vi "Lab Panel V5.25.vi"() -> ()   [LabVIEW 2017] (continued)
                      frame False {
                        # "update ambient referance temperature"
                        n2219 = case shown="True" w3927 {
                          tunnel: [w3929 100.0] -> w3928
                          frame False {
                            n2220 = local read "TEMP REF cal"() -> (w3929:dbl)
                          }
                          frame True {
                          }
                        }
                        n2221 = disable-structure shown="Disabled" {
                          frame Disabled {
                            n2222 = local read "Temp read loop"() -> ()  [unwired: 1 out]
                          }
                          frame Enabled {
                          }
                        }
                        n2223 = Multiply(x=w3928, y=w3926) -> (x*y=w3925:dbl)
                        n2224 = Subtract(x=w3925, y=272) -> (x-y=w3923:dbl)
                        "Amb Tp" <- w3923
                        n2225 = local write "Ref deg C"(w3923) -> ()
                        "deg C (volts)" <- w3926
                      }
                      frame True {
                      }
                    }
                  }
                }
              }
            }
          }
          frame #13 {
            # "save test data to file"
            n2226 = Get Date/Time In Seconds() -> (seconds since 1Jan1904=w3931:timestamp)
            "File Time Stamp" <- w3931
            n2227 = local read "on loops"() -> (w3950:dbl)
            n2228 = local read "jig cycle"() -> (w3947:dbl)
            n2229 = Format Date/Time String(time format string (%c)="%H:%M%:%S", seconds (now)=w3931) -> (date/time string=w3935:string)  [unwired: 1 in]
            n2230 = Add(x=w3950, y=2) -> (x+y=w3948:dbl)
            n2231 = Build Array(w3935) -> (w3934:string[])
            n2232 = Equal?(x=w3947, y=1) -> (x = y?=w3933:bool)
            n2233 = Equal?(x=w3947, y=w3948) -> (x = y?=w3932:bool)
            n2234 = stacked-sequence {
              tunnel: w3946 -> [w3956 _ _ _ _ _ _ _ _ _]
              tunnel: w3945 -> [_ w4032 _ _ _ _ _ _ _ _]
              tunnel: w3944 -> [_ _ w4112 _ _ _ _ _ _ _]
              tunnel: w3943 -> [_ _ _ w4192 _ _ _ _ _ _]
              tunnel: w3942 -> [_ _ _ _ w4272 _ _ _ _ _]
              tunnel: w3941 -> [_ _ _ _ _ w4352 _ _ _ _]
              tunnel: w3940 -> [_ _ _ _ _ _ w4432 _ _ _]
              tunnel: w3939 -> [_ _ _ _ _ _ _ w4512 _ _]
              tunnel: w3938 -> [_ _ _ _ _ _ _ _ w4592 _]
              tunnel: w3937 -> [_ _ _ _ _ _ _ _ _ w4672]
              tunnel: w3934 -> [w3955 w4036 w4116 w4196 w4276 w4356 w4436 w4516 w4596 w4676]
              tunnel: w3933 -> [w3954 w4035 w4115 w4195 w4275 w4355 w4435 w4515 w4595 w4675]
              tunnel: w3932 -> [w3953 w4034 w4114 w4194 w4274 w4354 w4434 w4514 w4594 w4674]
              tunnel: w3931 -> [w3952 w4033 w4113 w4193 w4273 w4353 w4433 w4513 w4593 w4673]
              frame #0 {
                n2235 = case shown="True" w3956 {
                  tunnel: w3955 -> [_ w3961]
                  tunnel: w3954 -> [_ w3960]
                  tunnel: w3953 -> [_ w3958]
                  tunnel: w3952 -> [_ w3957]
                  frame False {
                  }
                  frame True {
                    n2236 = local read "DISP LAB01-1"() -> (w3962:T4)
                    n2237 = local read "SIG LAB01-1"() -> (w3963:T2)
                    n2238 = local read "ON L01-1"() -> (w3959:cluster{"amps":dbl, "volts":dbl, "pf":dbl})
                    n2239 = Unbundle(w3963) -> ("AMPS"=w3969:dbl, "VOLTS"=w3967:dbl, "PF"=w3966:dbl, "Tmp Live"=w3965:dbl, "Tmp Neut"=w3968:dbl)
                    n2240 = Unbundle(w3962) -> ("CYCLE"=w3964:dbl)  [unwired: 2 out]
                    n2241 = stacked-sequence {
                      tunnel: w3969 -> [w3973 w3992]
                      tunnel: w3968 -> [_ w3991]
                      tunnel: w3967 -> [w3972 w3990]
                      tunnel: w3966 -> [w3971 w3989]
                      tunnel: w3965 -> [_ w3988]
                      tunnel: w3964 -> [_ w3987]
                      tunnel: w3961 -> [_ w3986]
                      tunnel: w3960 -> [w3974 _]
                      tunnel: w3959 -> [w3970 w3984]
                      tunnel: w3958 -> [_ w3985]
                      tunnel: w3957 -> [_ w3980]
                      frame #0 {
                        n2242 = case shown="True" w3974 {
                          tunnel: w3973 -> [_ w3979]
                          tunnel: w3972 -> [_ w3978]
                          tunnel: w3971 -> [_ w3977]
                          tunnel: w3970 -> [_ w3975]
                          frame False {
                          }
                          frame True {
                            n2243 = Bundle(cluster=w3975, "amps"=w3979, "volts"=w3978, "pf"=w3977) -> (w3976:cluster{"amps":dbl, "volts":dbl, "pf":dbl})
                            n2244 = local write "ON L01-1"(w3976) -> ()
                          }
                        }
                      }
                      frame #1 {
                        n2245 = Unbundle(w3984) -> ("amps"=w3983:dbl, "volts"=w3982:dbl, "pf"=w3981:dbl)
                        n2246 = case shown="True" w3985 {
                          tunnel: w3992 -> [_ w3993]
                          tunnel: w3991 -> [_ w4031]
                          tunnel: w3990 -> [_ _]
                          tunnel: w3989 -> [_ _]
                          tunnel: w3988 -> [_ w4030]
                          tunnel: w3987 -> [_ w4029]
                          tunnel: w3986 -> [_ w3997]
                          tunnel: w3983 -> [_ w3994]
                          tunnel: w3982 -> [_ w4026]
                          tunnel: w3981 -> [_ w4025]
                          tunnel: w3980 -> [_ w3995]
                          frame False {
                          }
                          frame True {
                            n2247 = local read "TDMS LAB01-1"() -> (w4028:refnum<k34>)
                            n2248 = Build Array(w4026) -> (w4022:dbl[])
                            n2249 = Build Array(w4025) -> (w4021:dbl[])
                            n2250 = Build Array(w4030) -> (w4020:dbl[])
                            n2251 = Build Array(w4031) -> (w4019:dbl[])
                            n2252 = Build Array(w3994) -> (w4024:dbl[])
                            n2253 = Build Array(w3993) -> (w4023:dbl[])
                            n2254 = Build Array(w4029) -> (w4018:dbl[])
                            n2255 = Build Array("AMPS ON", "AMPS OFF", "VOLTS", "PF", "TEMP Live", "TEMP Neut", "CYCLE") -> (w4002:string[])
                            n2256 = Bundle By Name("Y"=w4024, "t0"=w3995) -> (w4017:waveform(dbl))  [unwired: 1 in]
                            n2257 = Bundle By Name("Y"=w4023, "t0"=w3995) -> (w4016:waveform(dbl))  [unwired: 1 in]
                            n2258 = Bundle By Name("Y"=w4022, "t0"=w3995) -> (w4015:waveform(dbl))  [unwired: 1 in]
                            n2259 = Bundle By Name("Y"=w4021, "t0"=w3995) -> (w4014:waveform(dbl))  [unwired: 1 in]
                            n2260 = Bundle By Name("Y"=w4020, "t0"=w3995) -> (w4013:waveform(dbl))  [unwired: 1 in]
                            n2261 = Bundle By Name("Y"=w4019, "t0"=w3995) -> (w4012:waveform(dbl))  [unwired: 1 in]
                            n2262 = Bundle By Name("Y"=w4018, "t0"=w3995) -> (w4011:waveform(dbl))  [unwired: 1 in]
                            n2263 = Build Array(w4017, w4016, w4015, w4014, w4013, w4012, w4011) -> (w4010:waveform(dbl)[])
                            n2264 = TDMS Write(0:w4028, 5:"TEST VALUES", 7:w4002, 9:w4010) -> (4:w4001:refnum<k34>, 6:w4000:string, 15:w3999:errorcluster)  [unwired: 2 in, 1 out]
                            n2265 = TDMS Write(0:w4001, 5:w4000, 7:"TIME", 9:w3997, 11:w3999) -> (15:w3996:errorcluster)  [unwired: 1 in, 3 out]
                            n2266 = local write "data file error"(w3996) -> ()
                          }
                        }
                      }
                    }
                  }
                }
              }
              frame #1 {
                n2267 = case shown="True" w4032 {
                  tunnel: w4036 -> [_ w4041]
                  tunnel: w4035 -> [_ w4040]
                  tunnel: w4034 -> [_ w4038]
                  tunnel: w4033 -> [_ w4037]
                  frame False {
                  }
                  frame True {
                    n2268 = local read "DISP LAB01-2"() -> (w4042:T4)
                    n2269 = local read "SIG LAB01-2"() -> (w4043:T2)
                    n2270 = local read "ON L01-2"() -> (w4039:cluster{"amps":dbl, "volts":dbl, "pf":dbl})
                    n2271 = Unbundle(w4043) -> ("AMPS"=w4049:dbl, "VOLTS"=w4047:dbl, "PF"=w4046:dbl, "Tmp Live"=w4045:dbl, "Tmp Neut"=w4048:dbl)
                    n2272 = Unbundle(w4042) -> ("CYCLE"=w4044:dbl)  [unwired: 2 out]
                    n2273 = stacked-sequence {
                      tunnel: w4049 -> [w4053 w4072]
                      tunnel: w4048 -> [_ w4071]
                      tunnel: w4047 -> [w4052 w4070]
                      tunnel: w4046 -> [w4051 w4069]
                      tunnel: w4045 -> [_ w4068]
                      tunnel: w4044 -> [_ w4067]
                      tunnel: w4041 -> [_ w4066]
                      tunnel: w4040 -> [w4054 _]
                      tunnel: w4039 -> [w4050 w4064]
                      tunnel: w4038 -> [_ w4065]
                      tunnel: w4037 -> [_ w4060]
                      frame #0 {
                        n2274 = case shown="True" w4054 {
                          tunnel: w4053 -> [_ w4059]
                          tunnel: w4052 -> [_ w4058]
                          tunnel: w4051 -> [_ w4057]
                          tunnel: w4050 -> [_ w4055]
                          frame False {
                          }
                          frame True {
                            n2275 = Bundle(cluster=w4055, "amps"=w4059, "volts"=w4058, "pf"=w4057) -> (w4056:cluster{"amps":dbl, "volts":dbl, "pf":dbl})
                            n2276 = local write "ON L01-2"(w4056) -> ()
                          }
                        }
                      }
                      frame #1 {
                        n2277 = Unbundle(w4064) -> ("amps"=w4063:dbl, "volts"=w4062:dbl, "pf"=w4061:dbl)
                        n2278 = case shown="True" w4065 {
                          tunnel: w4072 -> [_ w4104]
                          tunnel: w4071 -> [_ w4111]
                          tunnel: w4070 -> [_ _]
                          tunnel: w4069 -> [_ _]
                          tunnel: w4068 -> [_ w4110]
                          tunnel: w4067 -> [_ w4109]
                          tunnel: w4066 -> [_ w4074]
                          tunnel: w4063 -> [_ w4106]
                          tunnel: w4062 -> [_ w4105]
                          tunnel: w4061 -> [_ w4103]
                          tunnel: w4060 -> [_ w4095]
                          frame False {
                          }
                          frame True {
                            n2279 = local read "TDMS LAB01-2"() -> (w4108:refnum<k34>)
                            n2280 = Build Array(w4105) -> (w4100:dbl[])
                            n2281 = Build Array(w4103) -> (w4099:dbl[])
                            n2282 = Build Array(w4110) -> (w4098:dbl[])
                            n2283 = Build Array(w4111) -> (w4097:dbl[])
                            n2284 = Build Array(w4106) -> (w4102:dbl[])
                            n2285 = Build Array(w4104) -> (w4101:dbl[])
                            n2286 = Build Array(w4109) -> (w4096:dbl[])
                            n2287 = Build Array("AMPS ON", "AMPS OFF", "VOLTS", "PF", "TEMP Live", "TEMP Neut", "CYCLE") -> (w4079:string[])
                            n2288 = Bundle By Name("Y"=w4102, "t0"=w4095) -> (w4094:waveform(dbl))  [unwired: 1 in]
                            n2289 = Bundle By Name("Y"=w4101, "t0"=w4095) -> (w4093:waveform(dbl))  [unwired: 1 in]
                            n2290 = Bundle By Name("Y"=w4100, "t0"=w4095) -> (w4092:waveform(dbl))  [unwired: 1 in]
                            n2291 = Bundle By Name("Y"=w4099, "t0"=w4095) -> (w4091:waveform(dbl))  [unwired: 1 in]
                            n2292 = Bundle By Name("Y"=w4098, "t0"=w4095) -> (w4090:waveform(dbl))  [unwired: 1 in]
                            n2293 = Bundle By Name("Y"=w4097, "t0"=w4095) -> (w4089:waveform(dbl))  [unwired: 1 in]
                            n2294 = Bundle By Name("Y"=w4096, "t0"=w4095) -> (w4088:waveform(dbl))  [unwired: 1 in]
                            n2295 = Build Array(w4094, w4093, w4092, w4091, w4090, w4089, w4088) -> (w4087:waveform(dbl)[])
                            n2296 = TDMS Write(0:w4108, 5:"TEST VALUES", 7:w4079, 9:w4087) -> (4:w4078:refnum<k34>, 6:w4077:string, 15:w4076:errorcluster)  [unwired: 2 in, 1 out]
                            n2297 = TDMS Write(0:w4078, 5:w4077, 7:"TIME", 9:w4074, 11:w4076) -> (15:w4073:errorcluster)  [unwired: 1 in, 3 out]
                            n2298 = local write "data file error"(w4073) -> ()
                          }
                        }
                      }
                    }
                  }
                }
              }
              frame #2 {
                n2299 = case shown="True" w4112 {
                  tunnel: w4116 -> [_ w4121]
                  tunnel: w4115 -> [_ w4120]
                  tunnel: w4114 -> [_ w4118]
                  tunnel: w4113 -> [_ w4117]
                  frame False {
                  }
                  frame True {
                    n2300 = local read "DISP LAB02-1"() -> (w4122:T4)
                    n2301 = local read "SIG LAB02-1"() -> (w4123:T2)
                    n2302 = local read "ON L02-1"() -> (w4119:cluster{"amps":dbl, "volts":dbl, "pf":dbl})
                    n2303 = Unbundle(w4123) -> ("AMPS"=w4129:dbl, "VOLTS"=w4127:dbl, "PF"=w4126:dbl, "Tmp Live"=w4125:dbl, "Tmp Neut"=w4128:dbl)
                    n2304 = Unbundle(w4122) -> ("CYCLE"=w4124:dbl)  [unwired: 2 out]
                    n2305 = stacked-sequence {
                      tunnel: w4129 -> [w4133 w4152]
                      tunnel: w4128 -> [_ w4151]
                      tunnel: w4127 -> [w4132 w4150]
                      tunnel: w4126 -> [w4131 w4149]
                      tunnel: w4125 -> [_ w4148]
                      tunnel: w4124 -> [_ w4147]
                      tunnel: w4121 -> [_ w4146]
                      tunnel: w4120 -> [w4134 _]
                      tunnel: w4119 -> [w4130 w4144]
                      tunnel: w4118 -> [_ w4145]
                      tunnel: w4117 -> [_ w4140]
                      frame #0 {
                        n2306 = case shown="True" w4134 {
                          tunnel: w4133 -> [_ w4139]
                          tunnel: w4132 -> [_ w4138]
                          tunnel: w4131 -> [_ w4137]
                          tunnel: w4130 -> [_ w4135]
                          frame False {
                          }
                          frame True {
                            n2307 = Bundle(cluster=w4135, "amps"=w4139, "volts"=w4138, "pf"=w4137) -> (w4136:cluster{"amps":dbl, "volts":dbl, "pf":dbl})
                            n2308 = local write "ON L02-1"(w4136) -> ()
                          }
                        }
                      }
                      frame #1 {
                        n2309 = Unbundle(w4144) -> ("amps"=w4143:dbl, "volts"=w4142:dbl, "pf"=w4141:dbl)
                        n2310 = case shown="True" w4145 {
                          tunnel: w4152 -> [_ w4184]
                          tunnel: w4151 -> [_ w4191]
                          tunnel: w4150 -> [_ _]
                          tunnel: w4149 -> [_ _]
                          tunnel: w4148 -> [_ w4190]
                          tunnel: w4147 -> [_ w4189]
                          tunnel: w4146 -> [_ w4154]
                          tunnel: w4143 -> [_ w4186]
                          tunnel: w4142 -> [_ w4185]
                          tunnel: w4141 -> [_ w4183]
                          tunnel: w4140 -> [_ w4175]
                          frame False {
                          }
                          frame True {
                            n2311 = local read "TDMS LAB02-1"() -> (w4188:refnum<k34>)
                            n2312 = Build Array(w4185) -> (w4180:dbl[])
                            n2313 = Build Array(w4183) -> (w4179:dbl[])
                            n2314 = Build Array(w4190) -> (w4178:dbl[])
                            n2315 = Build Array(w4191) -> (w4177:dbl[])
                            n2316 = Build Array(w4186) -> (w4182:dbl[])
                            n2317 = Build Array(w4184) -> (w4181:dbl[])
                            n2318 = Build Array(w4189) -> (w4176:dbl[])
                            n2319 = Build Array("AMPS ON", "AMPS OFF", "VOLTS", "PF", "TEMP Live", "TEMP Neut", "CYCLE") -> (w4159:string[])
                            n2320 = Bundle By Name("Y"=w4182, "t0"=w4175) -> (w4174:waveform(dbl))  [unwired: 1 in]
                            n2321 = Bundle By Name("Y"=w4181, "t0"=w4175) -> (w4173:waveform(dbl))  [unwired: 1 in]
                            n2322 = Bundle By Name("Y"=w4180, "t0"=w4175) -> (w4172:waveform(dbl))  [unwired: 1 in]
                            n2323 = Bundle By Name("Y"=w4179, "t0"=w4175) -> (w4171:waveform(dbl))  [unwired: 1 in]
                            n2324 = Bundle By Name("Y"=w4178, "t0"=w4175) -> (w4170:waveform(dbl))  [unwired: 1 in]
                            n2325 = Bundle By Name("Y"=w4177, "t0"=w4175) -> (w4169:waveform(dbl))  [unwired: 1 in]
                            n2326 = Bundle By Name("Y"=w4176, "t0"=w4175) -> (w4168:waveform(dbl))  [unwired: 1 in]
                            n2327 = Build Array(w4174, w4173, w4172, w4171, w4170, w4169, w4168) -> (w4167:waveform(dbl)[])
                            n2328 = TDMS Write(0:w4188, 5:"TEST VALUES", 7:w4159, 9:w4167) -> (4:w4158:refnum<k34>, 6:w4157:string, 15:w4156:errorcluster)  [unwired: 2 in, 1 out]
                            n2329 = TDMS Write(0:w4158, 5:w4157, 7:"TIME", 9:w4154, 11:w4156) -> (15:w4153:errorcluster)  [unwired: 1 in, 3 out]
                            n2330 = local write "data file error"(w4153) -> ()
                          }
                        }
                      }
                    }
                  }
                }
              }
              frame #3 {
                n2331 = case shown="True" w4192 {
                  tunnel: w4196 -> [_ w4201]
                  tunnel: w4195 -> [_ w4200]
                  tunnel: w4194 -> [_ w4198]
                  tunnel: w4193 -> [_ w4197]
                  frame False {
                  }
                  frame True {
                    n2332 = local read "DISP LAB02-2"() -> (w4202:T4)
                    n2333 = local read "SIG LAB02-2"() -> (w4203:T2)
                    n2334 = local read "ON L02-2"() -> (w4199:cluster{"amps":dbl, "volts":dbl, "pf":dbl})
                    n2335 = Unbundle(w4203) -> ("AMPS"=w4209:dbl, "VOLTS"=w4207:dbl, "PF"=w4206:dbl, "Tmp Live"=w4205:dbl, "Tmp Neut"=w4208:dbl)
                    n2336 = Unbundle(w4202) -> ("CYCLE"=w4204:dbl)  [unwired: 2 out]
                    n2337 = stacked-sequence {
                      tunnel: w4209 -> [w4213 w4232]
                      tunnel: w4208 -> [_ w4231]
                      tunnel: w4207 -> [w4212 w4230]
                      tunnel: w4206 -> [w4211 w4229]
                      tunnel: w4205 -> [_ w4228]
                      tunnel: w4204 -> [_ w4227]
                      tunnel: w4201 -> [_ w4226]
                      tunnel: w4200 -> [w4214 _]
                      tunnel: w4199 -> [w4210 w4224]
                      tunnel: w4198 -> [_ w4225]
                      tunnel: w4197 -> [_ w4220]
                      frame #0 {
                        n2338 = case shown="True" w4214 {
                          tunnel: w4213 -> [_ w4219]
                          tunnel: w4212 -> [_ w4218]
                          tunnel: w4211 -> [_ w4217]
                          tunnel: w4210 -> [_ w4215]
                          frame False {
                          }
                          frame True {
                            n2339 = Bundle(cluster=w4215, "amps"=w4219, "volts"=w4218, "pf"=w4217) -> (w4216:cluster{"amps":dbl, "volts":dbl, "pf":dbl})
                            n2340 = local write "ON L02-2"(w4216) -> ()
                          }
                        }
                      }
                      frame #1 {
                        n2341 = Unbundle(w4224) -> ("amps"=w4223:dbl, "volts"=w4222:dbl, "pf"=w4221:dbl)
                        n2342 = case shown="True" w4225 {
                          tunnel: w4232 -> [_ w4264]
                          tunnel: w4231 -> [_ w4271]
                          tunnel: w4230 -> [_ _]
                          tunnel: w4229 -> [_ _]
                          tunnel: w4228 -> [_ w4270]
                          tunnel: w4227 -> [_ w4269]
                          tunnel: w4226 -> [_ w4234]
                          tunnel: w4223 -> [_ w4266]
                          tunnel: w4222 -> [_ w4265]
                          tunnel: w4221 -> [_ w4263]
                          tunnel: w4220 -> [_ w4255]
                          frame False {
                          }
                          frame True {
                            n2343 = local read "TDMS LAB02-2"() -> (w4268:refnum<k34>)
                            n2344 = Build Array(w4265) -> (w4260:dbl[])
                            n2345 = Build Array(w4263) -> (w4259:dbl[])
                            n2346 = Build Array(w4270) -> (w4258:dbl[])
                            n2347 = Build Array(w4271) -> (w4257:dbl[])
                            n2348 = Build Array(w4266) -> (w4262:dbl[])
                            n2349 = Build Array(w4264) -> (w4261:dbl[])
                            n2350 = Build Array(w4269) -> (w4256:dbl[])
                            n2351 = Build Array("AMPS ON", "AMPS OFF", "VOLTS", "PF", "TEMP Live", "TEMP Neut", "CYCLE") -> (w4239:string[])
                            n2352 = Bundle By Name("Y"=w4262, "t0"=w4255) -> (w4254:waveform(dbl))  [unwired: 1 in]
                            n2353 = Bundle By Name("Y"=w4261, "t0"=w4255) -> (w4253:waveform(dbl))  [unwired: 1 in]
                            n2354 = Bundle By Name("Y"=w4260, "t0"=w4255) -> (w4252:waveform(dbl))  [unwired: 1 in]
                            n2355 = Bundle By Name("Y"=w4259, "t0"=w4255) -> (w4251:waveform(dbl))  [unwired: 1 in]
                            n2356 = Bundle By Name("Y"=w4258, "t0"=w4255) -> (w4250:waveform(dbl))  [unwired: 1 in]
                            n2357 = Bundle By Name("Y"=w4257, "t0"=w4255) -> (w4249:waveform(dbl))  [unwired: 1 in]
                            n2358 = Bundle By Name("Y"=w4256, "t0"=w4255) -> (w4248:waveform(dbl))  [unwired: 1 in]
                            n2359 = Build Array(w4254, w4253, w4252, w4251, w4250, w4249, w4248) -> (w4247:waveform(dbl)[])
                            n2360 = TDMS Write(0:w4268, 5:"TEST VALUES", 7:w4239, 9:w4247) -> (4:w4238:refnum<k34>, 6:w4237:string, 15:w4236:errorcluster)  [unwired: 2 in, 1 out]
                            n2361 = TDMS Write(0:w4238, 5:w4237, 7:"TIME", 9:w4234, 11:w4236) -> (15:w4233:errorcluster)  [unwired: 1 in, 3 out]
                            n2362 = local write "data file error"(w4233) -> ()
                          }
                        }
                      }
                    }
                  }
                }
              }
              frame #4 {
                n2363 = case shown="True" w4272 {
                  tunnel: w4276 -> [_ w4281]
                  tunnel: w4275 -> [_ w4280]
                  tunnel: w4274 -> [_ w4278]
                  tunnel: w4273 -> [_ w4277]
                  frame False {
                  }
                  frame True {
                    n2364 = local read "DISP LAB03-1"() -> (w4282:T4)
                    n2365 = local read "SIG LAB03-1"() -> (w4283:T2)
                    n2366 = local read "ON L03-1"() -> (w4279:cluster{"amps":dbl, "volts":dbl, "pf":dbl})
                    n2367 = Unbundle(w4283) -> ("AMPS"=w4289:dbl, "VOLTS"=w4287:dbl, "PF"=w4286:dbl, "Tmp Live"=w4285:dbl, "Tmp Neut"=w4288:dbl)
                    n2368 = Unbundle(w4282) -> ("CYCLE"=w4284:dbl)  [unwired: 2 out]
                    n2369 = stacked-sequence {
                      tunnel: w4289 -> [w4293 w4312]
                      tunnel: w4288 -> [_ w4311]
                      tunnel: w4287 -> [w4292 w4310]
                      tunnel: w4286 -> [w4291 w4309]
                      tunnel: w4285 -> [_ w4308]
                      tunnel: w4284 -> [_ w4307]
                      tunnel: w4281 -> [_ w4306]
                      tunnel: w4280 -> [w4294 _]
                      tunnel: w4279 -> [w4290 w4304]
                      tunnel: w4278 -> [_ w4305]
                      tunnel: w4277 -> [_ w4300]
                      frame #0 {
                        n2370 = case shown="True" w4294 {
                          tunnel: w4293 -> [_ w4299]
                          tunnel: w4292 -> [_ w4298]
                          tunnel: w4291 -> [_ w4297]
                          tunnel: w4290 -> [_ w4295]
                          frame False {
                          }
                          frame True {
                            n2371 = Bundle(cluster=w4295, "amps"=w4299, "volts"=w4298, "pf"=w4297) -> (w4296:cluster{"amps":dbl, "volts":dbl, "pf":dbl})
                            n2372 = local write "ON L03-1"(w4296) -> ()
                          }
                        }
                      }
                      frame #1 {
                        n2373 = Unbundle(w4304) -> ("amps"=w4303:dbl, "volts"=w4302:dbl, "pf"=w4301:dbl)
                        n2374 = case shown="True" w4305 {
                          tunnel: w4312 -> [_ w4344]
                          tunnel: w4311 -> [_ w4351]
                          tunnel: w4310 -> [_ _]
                          tunnel: w4309 -> [_ _]
                          tunnel: w4308 -> [_ w4350]
                          tunnel: w4307 -> [_ w4349]
                          tunnel: w4306 -> [_ w4314]
                          tunnel: w4303 -> [_ w4346]
                          tunnel: w4302 -> [_ w4345]
                          tunnel: w4301 -> [_ w4343]
                          tunnel: w4300 -> [_ w4335]
                          frame False {
                          }
                          frame True {
                            n2375 = local read "TDMS LAB03-1"() -> (w4348:refnum<k34>)
                            n2376 = Build Array(w4345) -> (w4340:dbl[])
                            n2377 = Build Array(w4343) -> (w4339:dbl[])
                            n2378 = Build Array(w4350) -> (w4338:dbl[])
                            n2379 = Build Array(w4351) -> (w4337:dbl[])
                            n2380 = Build Array(w4346) -> (w4342:dbl[])
                            n2381 = Build Array(w4344) -> (w4341:dbl[])
                            n2382 = Build Array(w4349) -> (w4336:dbl[])
                            n2383 = Build Array("AMPS ON", "AMPS OFF", "VOLTS", "PF", "TEMP Live", "TEMP Neut", "CYCLE") -> (w4319:string[])
                            n2384 = Bundle By Name("Y"=w4342, "t0"=w4335) -> (w4334:waveform(dbl))  [unwired: 1 in]
                            n2385 = Bundle By Name("Y"=w4341, "t0"=w4335) -> (w4333:waveform(dbl))  [unwired: 1 in]
                            n2386 = Bundle By Name("Y"=w4340, "t0"=w4335) -> (w4332:waveform(dbl))  [unwired: 1 in]
                            n2387 = Bundle By Name("Y"=w4339, "t0"=w4335) -> (w4331:waveform(dbl))  [unwired: 1 in]
                            n2388 = Bundle By Name("Y"=w4338, "t0"=w4335) -> (w4330:waveform(dbl))  [unwired: 1 in]
                            n2389 = Bundle By Name("Y"=w4337, "t0"=w4335) -> (w4329:waveform(dbl))  [unwired: 1 in]
                            n2390 = Bundle By Name("Y"=w4336, "t0"=w4335) -> (w4328:waveform(dbl))  [unwired: 1 in]
                            n2391 = Build Array(w4334, w4333, w4332, w4331, w4330, w4329, w4328) -> (w4327:waveform(dbl)[])
                            n2392 = TDMS Write(0:w4348, 5:"TEST VALUES", 7:w4319, 9:w4327) -> (4:w4318:refnum<k34>, 6:w4317:string, 15:w4316:errorcluster)  [unwired: 2 in, 1 out]
                            n2393 = TDMS Write(0:w4318, 5:w4317, 7:"TIME", 9:w4314, 11:w4316) -> (15:w4313:errorcluster)  [unwired: 1 in, 3 out]
                            n2394 = local write "data file error"(w4313) -> ()
                          }
                        }
                      }
                    }
                  }
                }
              }
              frame #5 {
                n2395 = case shown="True" w4352 {
                  tunnel: w4356 -> [_ w4361]
                  tunnel: w4355 -> [_ w4360]
                  tunnel: w4354 -> [_ w4358]
                  tunnel: w4353 -> [_ w4357]
                  frame False {
                  }
                  frame True {
                    n2396 = local read "DISP LAB03-2"() -> (w4362:T4)
                    n2397 = local read "SIG LAB03-2"() -> (w4363:T2)
                    n2398 = local read "ON L03-2"() -> (w4359:cluster{"amps":dbl, "volts":dbl, "pf":dbl})
                    n2399 = Unbundle(w4363) -> ("AMPS"=w4369:dbl, "VOLTS"=w4367:dbl, "PF"=w4366:dbl, "Tmp Live"=w4365:dbl, "Tmp Neut"=w4368:dbl)
                    n2400 = Unbundle(w4362) -> ("CYCLE"=w4364:dbl)  [unwired: 2 out]
                    n2401 = stacked-sequence {
                      tunnel: w4369 -> [w4373 w4392]
                      tunnel: w4368 -> [_ w4391]
                      tunnel: w4367 -> [w4372 w4390]
                      tunnel: w4366 -> [w4371 w4389]
                      tunnel: w4365 -> [_ w4388]
                      tunnel: w4364 -> [_ w4387]
                      tunnel: w4361 -> [_ w4386]
                      tunnel: w4360 -> [w4374 _]
                      tunnel: w4359 -> [w4370 w4384]
                      tunnel: w4358 -> [_ w4385]
                      tunnel: w4357 -> [_ w4380]
                      frame #0 {
                        n2402 = case shown="True" w4374 {
                          tunnel: w4373 -> [_ w4379]
                          tunnel: w4372 -> [_ w4378]
                          tunnel: w4371 -> [_ w4377]
                          tunnel: w4370 -> [_ w4375]
                          frame False {
                          }
                          frame True {
                            n2403 = Bundle(cluster=w4375, "amps"=w4379, "volts"=w4378, "pf"=w4377) -> (w4376:cluster{"amps":dbl, "volts":dbl, "pf":dbl})
                            n2404 = local write "ON L03-2"(w4376) -> ()
                          }
                        }
                      }
                      frame #1 {
                        n2405 = Unbundle(w4384) -> ("amps"=w4383:dbl, "volts"=w4382:dbl, "pf"=w4381:dbl)
                        n2406 = case shown="True" w4385 {
                          tunnel: w4392 -> [_ w4424]
                          tunnel: w4391 -> [_ w4431]
                          tunnel: w4390 -> [_ _]
                          tunnel: w4389 -> [_ _]
                          tunnel: w4388 -> [_ w4430]
                          tunnel: w4387 -> [_ w4429]
                          tunnel: w4386 -> [_ w4394]
                          tunnel: w4383 -> [_ w4426]
                          tunnel: w4382 -> [_ w4425]
                          tunnel: w4381 -> [_ w4423]
                          tunnel: w4380 -> [_ w4415]
                          frame False {
                          }
                          frame True {
                            n2407 = local read "TDMS LAB03-2"() -> (w4428:refnum<k34>)
                            n2408 = Build Array(w4425) -> (w4420:dbl[])
                            n2409 = Build Array(w4423) -> (w4419:dbl[])
                            n2410 = Build Array(w4430) -> (w4418:dbl[])
                            n2411 = Build Array(w4431) -> (w4417:dbl[])
                            n2412 = Build Array(w4426) -> (w4422:dbl[])
                            n2413 = Build Array(w4424) -> (w4421:dbl[])
                            n2414 = Build Array(w4429) -> (w4416:dbl[])
                            n2415 = Build Array("AMPS ON", "AMPS OFF", "VOLTS", "PF", "TEMP Live", "TEMP Neut", "CYCLE") -> (w4399:string[])
                            n2416 = Bundle By Name("Y"=w4422, "t0"=w4415) -> (w4414:waveform(dbl))  [unwired: 1 in]
                            n2417 = Bundle By Name("Y"=w4421, "t0"=w4415) -> (w4413:waveform(dbl))  [unwired: 1 in]
                            n2418 = Bundle By Name("Y"=w4420, "t0"=w4415) -> (w4412:waveform(dbl))  [unwired: 1 in]
                            n2419 = Bundle By Name("Y"=w4419, "t0"=w4415) -> (w4411:waveform(dbl))  [unwired: 1 in]
                            n2420 = Bundle By Name("Y"=w4418, "t0"=w4415) -> (w4410:waveform(dbl))  [unwired: 1 in]
                            n2421 = Bundle By Name("Y"=w4417, "t0"=w4415) -> (w4409:waveform(dbl))  [unwired: 1 in]
                            n2422 = Bundle By Name("Y"=w4416, "t0"=w4415) -> (w4408:waveform(dbl))  [unwired: 1 in]
                            n2423 = Build Array(w4414, w4413, w4412, w4411, w4410, w4409, w4408) -> (w4407:waveform(dbl)[])
                            n2424 = TDMS Write(0:w4428, 5:"TEST VALUES", 7:w4399, 9:w4407) -> (4:w4398:refnum<k34>, 6:w4397:string, 15:w4396:errorcluster)  [unwired: 2 in, 1 out]
                            n2425 = TDMS Write(0:w4398, 5:w4397, 7:"TIME", 9:w4394, 11:w4396) -> (15:w4393:errorcluster)  [unwired: 1 in, 3 out]
                            n2426 = local write "data file error"(w4393) -> ()
                          }
                        }
                      }
                    }
                  }
                }
              }
              frame #6 {
                n2427 = case shown="True" w4432 {
                  tunnel: w4436 -> [_ w4441]
                  tunnel: w4435 -> [_ w4440]
                  tunnel: w4434 -> [_ w4438]
                  tunnel: w4433 -> [_ w4437]
                  frame False {
                  }
                  frame True {
                    n2428 = local read "DISP LAB04-1"() -> (w4442:T4)
                    n2429 = local read "SIG LAB04-1"() -> (w4443:T2)
                    n2430 = local read "ON L04-1"() -> (w4439:cluster{"amps":dbl, "volts":dbl, "pf":dbl})
                    n2431 = Unbundle(w4443) -> ("AMPS"=w4449:dbl, "VOLTS"=w4447:dbl, "PF"=w4446:dbl, "Tmp Live"=w4445:dbl, "Tmp Neut"=w4448:dbl)
                    n2432 = Unbundle(w4442) -> ("CYCLE"=w4444:dbl)  [unwired: 2 out]
                    n2433 = stacked-sequence {
                      tunnel: w4449 -> [w4453 w4472]
                      tunnel: w4448 -> [_ w4471]
                      tunnel: w4447 -> [w4452 w4470]
                      tunnel: w4446 -> [w4451 w4469]
                      tunnel: w4445 -> [_ w4468]
                      tunnel: w4444 -> [_ w4467]
                      tunnel: w4441 -> [_ w4466]
                      tunnel: w4440 -> [w4454 _]
                      tunnel: w4439 -> [w4450 w4464]
                      tunnel: w4438 -> [_ w4465]
                      tunnel: w4437 -> [_ w4460]
                      frame #0 {
                        n2434 = case shown="True" w4454 {
                          tunnel: w4453 -> [_ w4459]
                          tunnel: w4452 -> [_ w4458]
                          tunnel: w4451 -> [_ w4457]
                          tunnel: w4450 -> [_ w4455]
                          frame False {
                          }
                          frame True {
                            n2435 = Bundle(cluster=w4455, "amps"=w4459, "volts"=w4458, "pf"=w4457) -> (w4456:cluster{"amps":dbl, "volts":dbl, "pf":dbl})
                            n2436 = local write "ON L04-1"(w4456) -> ()
                          }
                        }
                      }
                      frame #1 {
                        n2437 = Unbundle(w4464) -> ("amps"=w4463:dbl, "volts"=w4462:dbl, "pf"=w4461:dbl)
                        n2438 = case shown="True" w4465 {
                          tunnel: w4472 -> [_ w4504]
                          tunnel: w4471 -> [_ w4511]
                          tunnel: w4470 -> [_ _]
                          tunnel: w4469 -> [_ _]
                          tunnel: w4468 -> [_ w4510]
                          tunnel: w4467 -> [_ w4509]
                          tunnel: w4466 -> [_ w4474]
                          tunnel: w4463 -> [_ w4506]
                          tunnel: w4462 -> [_ w4505]
                          tunnel: w4461 -> [_ w4503]
                          tunnel: w4460 -> [_ w4495]
                          frame False {
                          }
                          frame True {
                            n2439 = local read "TDMS LAB04-1"() -> (w4508:refnum<k34>)
                            n2440 = Build Array(w4505) -> (w4500:dbl[])
                            n2441 = Build Array(w4503) -> (w4499:dbl[])
                            n2442 = Build Array(w4510) -> (w4498:dbl[])
                            n2443 = Build Array(w4511) -> (w4497:dbl[])
                            n2444 = Build Array(w4506) -> (w4502:dbl[])
                            n2445 = Build Array(w4504) -> (w4501:dbl[])
                            n2446 = Build Array(w4509) -> (w4496:dbl[])
                            n2447 = Build Array("AMPS ON", "AMPS OFF", "VOLTS", "PF", "TEMP Live", "TEMP Neut", "CYCLE") -> (w4479:string[])
                            n2448 = Bundle By Name("Y"=w4502, "t0"=w4495) -> (w4494:waveform(dbl))  [unwired: 1 in]
                            n2449 = Bundle By Name("Y"=w4501, "t0"=w4495) -> (w4493:waveform(dbl))  [unwired: 1 in]
                            n2450 = Bundle By Name("Y"=w4500, "t0"=w4495) -> (w4492:waveform(dbl))  [unwired: 1 in]
                            n2451 = Bundle By Name("Y"=w4499, "t0"=w4495) -> (w4491:waveform(dbl))  [unwired: 1 in]
                            n2452 = Bundle By Name("Y"=w4498, "t0"=w4495) -> (w4490:waveform(dbl))  [unwired: 1 in]
                            n2453 = Bundle By Name("Y"=w4497, "t0"=w4495) -> (w4489:waveform(dbl))  [unwired: 1 in]
                            n2454 = Bundle By Name("Y"=w4496, "t0"=w4495) -> (w4488:waveform(dbl))  [unwired: 1 in]
                            n2455 = Build Array(w4494, w4493, w4492, w4491, w4490, w4489, w4488) -> (w4487:waveform(dbl)[])
                            n2456 = TDMS Write(0:w4508, 5:"TEST VALUES", 7:w4479, 9:w4487) -> (4:w4478:refnum<k34>, 6:w4477:string, 15:w4476:errorcluster)  [unwired: 2 in, 1 out]
                            n2457 = TDMS Write(0:w4478, 5:w4477, 7:"TIME", 9:w4474, 11:w4476) -> (15:w4473:errorcluster)  [unwired: 1 in, 3 out]
                            n2458 = local write "data file error"(w4473) -> ()
                          }
                        }
                      }
                    }
                  }
                }
              }
              frame #7 {
                n2459 = case shown="True" w4512 {
                  tunnel: w4516 -> [_ w4521]
                  tunnel: w4515 -> [_ w4520]
                  tunnel: w4514 -> [_ w4518]
                  tunnel: w4513 -> [_ w4517]
                  frame False {
                  }
                  frame True {
                    n2460 = local read "DISP LAB04-2"() -> (w4522:T4)
                    n2461 = local read "SIG LAB04-2"() -> (w4523:T2)
                    n2462 = local read "ON L04-2"() -> (w4519:cluster{"amps":dbl, "volts":dbl, "pf":dbl})
                    n2463 = Unbundle(w4523) -> ("AMPS"=w4529:dbl, "VOLTS"=w4527:dbl, "PF"=w4526:dbl, "Tmp Live"=w4525:dbl, "Tmp Neut"=w4528:dbl)
                    n2464 = Unbundle(w4522) -> ("CYCLE"=w4524:dbl)  [unwired: 2 out]
                    n2465 = stacked-sequence {
                      tunnel: w4529 -> [w4533 w4552]
                      tunnel: w4528 -> [_ w4551]
                      tunnel: w4527 -> [w4532 w4550]
                      tunnel: w4526 -> [w4531 w4549]
                      tunnel: w4525 -> [_ w4548]
                      tunnel: w4524 -> [_ w4547]
                      tunnel: w4521 -> [_ w4546]
                      tunnel: w4520 -> [w4534 _]
                      tunnel: w4519 -> [w4530 w4544]
                      tunnel: w4518 -> [_ w4545]
                      tunnel: w4517 -> [_ w4540]
                      frame #0 {
                        n2466 = case shown="True" w4534 {
                          tunnel: w4533 -> [_ w4539]
                          tunnel: w4532 -> [_ w4538]
                          tunnel: w4531 -> [_ w4537]
                          tunnel: w4530 -> [_ w4535]
                          frame False {
                          }
                          frame True {
                            n2467 = Bundle(cluster=w4535, "amps"=w4539, "volts"=w4538, "pf"=w4537) -> (w4536:cluster{"amps":dbl, "volts":dbl, "pf":dbl})
                            n2468 = local write "ON L04-2"(w4536) -> ()
                          }
                        }
                      }
                      frame #1 {
                        n2469 = Unbundle(w4544) -> ("amps"=w4543:dbl, "volts"=w4542:dbl, "pf"=w4541:dbl)
                        n2470 = case shown="True" w4545 {
                          tunnel: w4552 -> [_ w4584]
                          tunnel: w4551 -> [_ w4591]
                          tunnel: w4550 -> [_ _]
                          tunnel: w4549 -> [_ _]
                          tunnel: w4548 -> [_ w4590]
                          tunnel: w4547 -> [_ w4589]
                          tunnel: w4546 -> [_ w4554]
                          tunnel: w4543 -> [_ w4586]
                          tunnel: w4542 -> [_ w4585]
                          tunnel: w4541 -> [_ w4583]
                          tunnel: w4540 -> [_ w4575]
                          frame False {
                          }
                          frame True {
                            n2471 = local read "TDMS LAB04-2"() -> (w4588:refnum<k34>)
                            n2472 = Build Array(w4585) -> (w4580:dbl[])
                            n2473 = Build Array(w4583) -> (w4579:dbl[])
                            n2474 = Build Array(w4590) -> (w4578:dbl[])
                            n2475 = Build Array(w4591) -> (w4577:dbl[])
                            n2476 = Build Array(w4586) -> (w4582:dbl[])
                            n2477 = Build Array(w4584) -> (w4581:dbl[])
                            n2478 = Build Array(w4589) -> (w4576:dbl[])
                            n2479 = Build Array("AMPS ON", "AMPS OFF", "VOLTS", "PF", "TEMP Live", "TEMP Neut", "CYCLE") -> (w4559:string[])
                            n2480 = Bundle By Name("Y"=w4582, "t0"=w4575) -> (w4574:waveform(dbl))  [unwired: 1 in]
                            n2481 = Bundle By Name("Y"=w4581, "t0"=w4575) -> (w4573:waveform(dbl))  [unwired: 1 in]
                            n2482 = Bundle By Name("Y"=w4580, "t0"=w4575) -> (w4572:waveform(dbl))  [unwired: 1 in]
                            n2483 = Bundle By Name("Y"=w4579, "t0"=w4575) -> (w4571:waveform(dbl))  [unwired: 1 in]
                            n2484 = Bundle By Name("Y"=w4578, "t0"=w4575) -> (w4570:waveform(dbl))  [unwired: 1 in]
                            n2485 = Bundle By Name("Y"=w4577, "t0"=w4575) -> (w4569:waveform(dbl))  [unwired: 1 in]
                            n2486 = Bundle By Name("Y"=w4576, "t0"=w4575) -> (w4568:waveform(dbl))  [unwired: 1 in]
                            n2487 = Build Array(w4574, w4573, w4572, w4571, w4570, w4569, w4568) -> (w4567:waveform(dbl)[])
                            n2488 = TDMS Write(0:w4588, 5:"TEST VALUES", 7:w4559, 9:w4567) -> (4:w4558:refnum<k34>, 6:w4557:string, 15:w4556:errorcluster)  [unwired: 2 in, 1 out]
                            n2489 = TDMS Write(0:w4558, 5:w4557, 7:"TIME", 9:w4554, 11:w4556) -> (15:w4553:errorcluster)  [unwired: 1 in, 3 out]
                            n2490 = local write "data file error"(w4553) -> ()
                          }
                        }
                      }
                    }
                  }
                }
              }
              frame #8 {
                n2491 = case shown="True" w4592 {
                  tunnel: w4596 -> [_ w4601]
                  tunnel: w4595 -> [_ w4600]
                  tunnel: w4594 -> [_ w4598]
                  tunnel: w4593 -> [_ w4597]
                  frame False {
                  }
                  frame True {
                    n2492 = local read "DISP LAB05-1"() -> (w4602:T4)
                    n2493 = local read "SIG LAB05-1"() -> (w4603:T2)
                    n2494 = local read "ON L05-1"() -> (w4599:cluster{"amps":dbl, "volts":dbl, "pf":dbl})
                    n2495 = Unbundle(w4603) -> ("AMPS"=w4609:dbl, "VOLTS"=w4607:dbl, "PF"=w4606:dbl, "Tmp Live"=w4605:dbl, "Tmp Neut"=w4608:dbl)
                    n2496 = Unbundle(w4602) -> ("CYCLE"=w4604:dbl)  [unwired: 2 out]
                    n2497 = stacked-sequence {
                      tunnel: w4609 -> [w4613 w4632]
                      tunnel: w4608 -> [_ w4631]
                      tunnel: w4607 -> [w4612 w4630]
                      tunnel: w4606 -> [w4611 w4629]
                      tunnel: w4605 -> [_ w4628]
                      tunnel: w4604 -> [_ w4627]
                      tunnel: w4601 -> [_ w4626]
                      tunnel: w4600 -> [w4614 _]
                      tunnel: w4599 -> [w4610 w4624]
                      tunnel: w4598 -> [_ w4625]
                      tunnel: w4597 -> [_ w4620]
                      frame #0 {
                        n2498 = case shown="True" w4614 {
                          tunnel: w4613 -> [_ w4619]
                          tunnel: w4612 -> [_ w4618]
                          tunnel: w4611 -> [_ w4617]
                          tunnel: w4610 -> [_ w4615]
                          frame False {
                          }
                          frame True {
                            n2499 = Bundle(cluster=w4615, "amps"=w4619, "volts"=w4618, "pf"=w4617) -> (w4616:cluster{"amps":dbl, "volts":dbl, "pf":dbl})
                            n2500 = local write "ON L05-1"(w4616) -> ()
                          }
                        }
                      }
                      frame #1 {
                        n2501 = Unbundle(w4624) -> ("amps"=w4623:dbl, "volts"=w4622:dbl, "pf"=w4621:dbl)
                        n2502 = case shown="True" w4625 {
                          tunnel: w4632 -> [_ w4664]
                          tunnel: w4631 -> [_ w4671]
                          tunnel: w4630 -> [_ _]
                          tunnel: w4629 -> [_ _]
                          tunnel: w4628 -> [_ w4670]
                          tunnel: w4627 -> [_ w4669]
                          tunnel: w4626 -> [_ w4634]
                          tunnel: w4623 -> [_ w4666]
                          tunnel: w4622 -> [_ w4665]
                          tunnel: w4621 -> [_ w4663]
                          tunnel: w4620 -> [_ w4655]
                          frame False {
                          }
                          frame True {
                            n2503 = local read "TDMS LAB05-1"() -> (w4668:refnum<k34>)
                            n2504 = Build Array(w4665) -> (w4660:dbl[])
                            n2505 = Build Array(w4663) -> (w4659:dbl[])
                            n2506 = Build Array(w4670) -> (w4658:dbl[])
                            n2507 = Build Array(w4671) -> (w4657:dbl[])
                            n2508 = Build Array(w4666) -> (w4662:dbl[])
                            n2509 = Build Array(w4664) -> (w4661:dbl[])
                            n2510 = Build Array(w4669) -> (w4656:dbl[])
                            n2511 = Build Array("AMPS ON", "AMPS OFF", "VOLTS", "PF", "TEMP Live", "TEMP Neut", "CYCLE") -> (w4639:string[])
                            n2512 = Bundle By Name("Y"=w4662, "t0"=w4655) -> (w4654:waveform(dbl))  [unwired: 1 in]
                            n2513 = Bundle By Name("Y"=w4661, "t0"=w4655) -> (w4653:waveform(dbl))  [unwired: 1 in]
                            n2514 = Bundle By Name("Y"=w4660, "t0"=w4655) -> (w4652:waveform(dbl))  [unwired: 1 in]
                            n2515 = Bundle By Name("Y"=w4659, "t0"=w4655) -> (w4651:waveform(dbl))  [unwired: 1 in]
                            n2516 = Bundle By Name("Y"=w4658, "t0"=w4655) -> (w4650:waveform(dbl))  [unwired: 1 in]
                            n2517 = Bundle By Name("Y"=w4657, "t0"=w4655) -> (w4649:waveform(dbl))  [unwired: 1 in]
                            n2518 = Bundle By Name("Y"=w4656, "t0"=w4655) -> (w4648:waveform(dbl))  [unwired: 1 in]
                            n2519 = Build Array(w4654, w4653, w4652, w4651, w4650, w4649, w4648) -> (w4647:waveform(dbl)[])
                            n2520 = TDMS Write(0:w4668, 5:"TEST VALUES", 7:w4639, 9:w4647) -> (4:w4638:refnum<k34>, 6:w4637:string, 15:w4636:errorcluster)  [unwired: 2 in, 1 out]
                            n2521 = TDMS Write(0:w4638, 5:w4637, 7:"TIME", 9:w4634, 11:w4636) -> (15:w4633:errorcluster)  [unwired: 1 in, 3 out]
                            n2522 = local write "data file error"(w4633) -> ()
                          }
                        }
                      }
                    }
                  }
                }
